vi "Rh_to_Absolute_Humidity.vi"(1 "Temperature (C)":dbl, 2 "Relative Humidity":dbl) -> (0 "Absolute Humidity":dbl)   [LabVIEW 2020]
doc: "Converts relative humidity (xx%) to absolute humidity, using the system temperature in celsius."
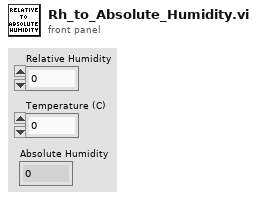
[diagram p1: front panel]
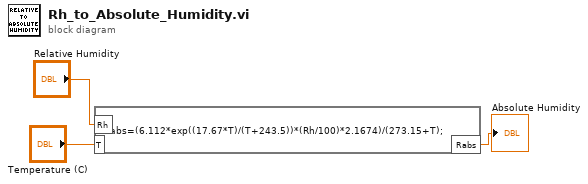
[diagram p0: block diagram]
diagram:
  n1 = formula code="Rabs=(6.112*exp((17.67*T)/(T+243.5))*(Rh/100)*2.1674)/(273.15+T);"("Rh"="Relative Humidity", "T"="Temperature (C)") -> ("Rabs"=→"Absolute Humidity":dbl)
